vi "SP Format CH Traces.vi"(7 "Limit Traces":T5(array[cluster]), 8 "error in (no error)":errorcluster, 9 "CH2 Controls":T1={"Trace On"=TRUE, "Measure"=0, "Format"=0, "Autoscale"=TRUE, "Reference"=0.0, "\nRefUnit"="dB/Div", "Position"=5.0, "Scale"=10.0, "ScaleUnit"="dB/Div", "LimitOn"=TRUE, "LimitFill"=FALSE, "Display Data"=0, "Show Markers"=TRUE, "SXX"=""} {"Reference" format="%#.2g"; "Display Data" items=["Data", "Memory", "Data/Memory"]; "Format" items=["Log Mag", "Phase", "Expanded Phase", "Delay", "Smith", "Polar", "Lin Mag", "SWR", "Loss", "Real", "Imaginary"]; "Scale" min=0.001 step=1.0 format="%#.2g"; "Position" min=0.0 max=10.0}, 10 "CH1 Controls":T1={"Trace On"=TRUE, "Measure"=0, "Format"=0, "Autoscale"=TRUE, "Reference"=0.0, "\nRefUnit"="dB/Div", "Position"=5.0, "Scale"=10.0, "ScaleUnit"="dB/Div", "LimitOn"=TRUE, "LimitFill"=FALSE, "Display Data"=0, "Show Markers"=TRUE, "SXX"=""} {"Reference" format="%#.2g"; "Display Data" items=["Data", "Memory", "Data/Memory"]; "Format" items=["Log Mag", "Phase", "Expanded Phase", "Delay", "Smith", "Polar", "Lin Mag", "SWR", "Loss", "Real", "Imaginary"]; "Scale" min=0.001 step=1.0 format="%#.2g"; "Position" min=0.0 max=10.0}, 11 "Plot Reference":refnum<vi>) -> (0 "error out":errorcluster, 3 "Plot Reference":refnum<vi>)   [LabVIEW 2011]
uses:
  TypeDefs/SP Limit Type.ctl
  TypeDefs/SP Display Trace Controls.ctl
  TypeDefs/SP Display Format.ctl
  TypeDefs/SP Display Data.ctl
panel:
  # "Div"
  # "Div"
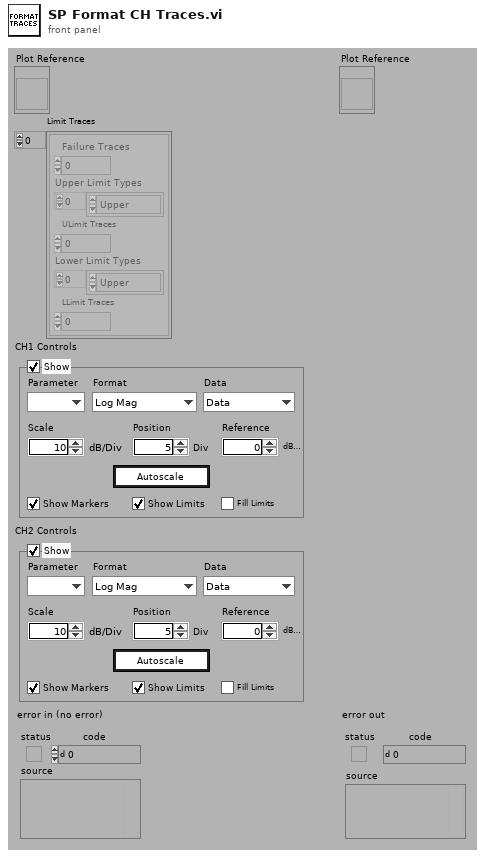
[diagram p1: front panel]
types:
  T1 = typedef "SP Display Trace Controls.ctl" = cluster{"Trace On":bool, "Measure":i32, "Format":T2, "Autoscale":bool, "Reference":dbl, "\nRefUnit":string, "Position":dbl, "Scale":dbl, "ScaleUnit":string, "LimitOn":bool, "LimitFill":bool, "Display Data":T3, "Show Markers":bool, "SXX":string}
  T2 = typedef "SP Display Format.ctl" = i32
  T3 = typedef "SP Display Data.ctl" = u16
  T4 = typedef "SP Limit Type.ctl" = enum16{"Upper", "Lower", "Delta", "Filter", "Referential"}
  T5 = cluster{"Failure Traces":i32, "Upper Limit Types":T4[], "ULimit Traces":i32, "Lower Limit Types":T4[], "LLimit Traces":i32}[]
  T6 = cluster{"Failure Traces":i32, "Upper Limit Types":T4[], "ULimit Traces":i32, "Lower Limit Types":T4[], "LLimit Traces":i32}
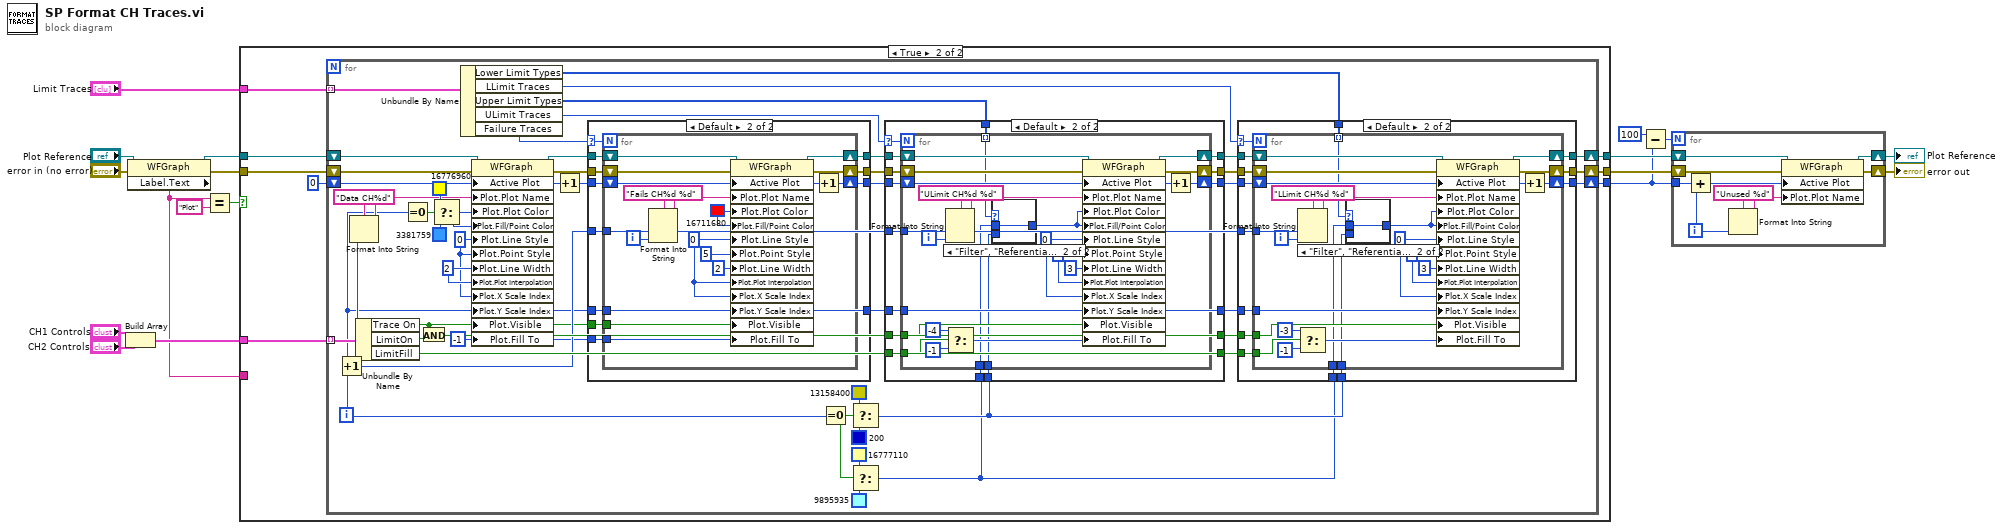
[diagram p0: block diagram]
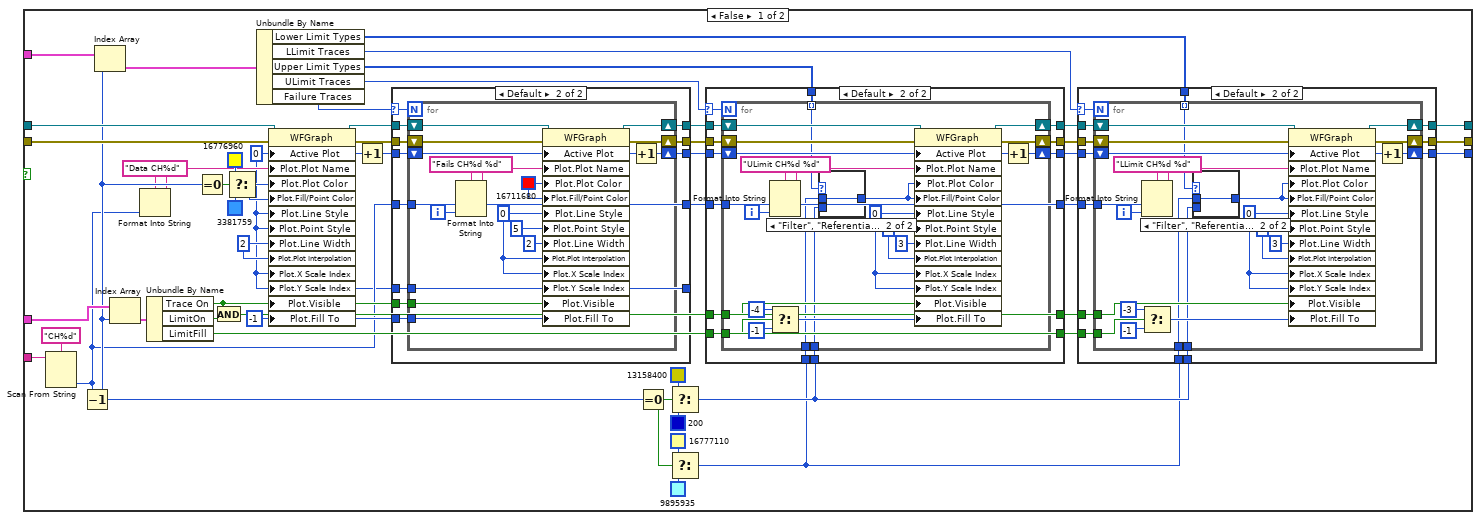
[diagram p2: hidden frame]
diagram:
  n1 = Build Array("CH1 Controls", "CH2 Controls") -> (w9:T1[])
  n2 = property on="Property Node" class="WFGraph"(reference="Plot Reference", error in="error in (no error)") -> (reference out=w14:refnum<vi>, error out=w16:errorcluster, "Label.Text"=w1:string)
  n3 = Equal?(x=w1, y="Plot") -> (x = y?=w12:bool)
  n4 = case shown="True" w12 {
    tunnel: [w50 w193] -> w7
    tunnel: [w51 w190] -> w8
    tunnel: "Limit Traces" -> [w67 w189]
    tunnel: w16 -> [w65 w192]
    tunnel: w14 -> [w64 w191]
    tunnel: w9 -> [w58 w187]
    tunnel: [w19 w186] -> w2
    tunnel: w1 -> [w41 _]
    frame False {
      w36 = i16 -1 ("Plot.Fill To")
      w59 = u8 2 ("Plot.Line Style")
      w21 = u32 0 ("Active Plot")
      n5 = Scan From String(format string="CH%d", input string=w41) -> (output 1=w33:i32)  [unwired: 2 in, 4 out]
      n6 = Decrement(x=w33) -> (x-1=w45:i32)
      n7 = Index Array(array=w67, index=w45) -> (element=w66:T6)
      n8 = Index Array(array=w58, index=w45) -> (element=w57:T1)
      n9 = Format Into String(format string="Data CH%d" ("Plot.Plot Name"), w33) -> (resulting string=w43:string)  [unwired: 2 in, 1 out]
      n10 = Unbundle By Name(w57) -> ("Trace On"=w37:bool, "LimitOn"=w56:bool, "LimitFill"=w48:bool)
      n11 = Equal To 0?(x=w45) -> (x = 0?=w61:bool)
      n12 = And(x=w37, y=w56) -> (x .and. y?=w47:bool)
      n13 = Select(t=u32 16776960, s=w61, f=u32 3381759) -> (s? t:f=w60:u32)
      n14 = Unbundle By Name(w66) -> ("Lower Limit Types"=w27:T4[], "LLimit Traces"=w52:i32, "Upper Limit Types"=w26:T4[], "ULimit Traces"=w55:i32, "Failure Traces"=w28:i32)
      n15 = property on="Property Node" class="WFGraph"(reference=w64, error in=w65, "Active Plot"=w21, "Plot.Plot Name"=w43, "Plot.Plot Color"=w60, "Plot.Fill/Point Color"=w60, "Plot.Line Style"=w21, "Plot.Point Style"=w21, "Plot.Line Width"=w59, "Plot.Plot Interpolation"=w59, "Plot.X Scale Index"=w21, "Plot.Y Scale Index"=w21, "Plot.Visible"=w37, "Plot.Fill To"=w36) -> (reference out=w30:refnum<vi>, error out=w29:errorcluster)
      n16 = Increment(x=w21) -> (x+1=w20:u32)
      n17 = case shown="Default" w28 {
        selector: w28 -> [_ w82]
        tunnel: [w74 w85] -> w38
        tunnel: [w73 w84] -> w39
        tunnel: [w72 w83] -> w40
        tunnel: w33 -> [w70 w76]
        tunnel: w20 -> [w74 w75]
        tunnel: w30 -> [w72 w81]
        tunnel: w29 -> [w73 w80]
        tunnel: w37 -> [_ w79]
        tunnel: w36 -> [_ w78]
        tunnel: w21 -> [w71 w77]
        tunnel: [w71 w77] -> _
        tunnel: [w70 w76] -> w32
        frame 0 {
        }
        frame Default {
          n18 = for {
            N: w82 -> [_]
            shift-right: [w100] -> w84
            shift-left: w80 -> [w101]
            shift-right: [w96] -> w83
            shift-left: w81 -> [w102]
            tunnel: w76 -> [w93]
            tunnel: w79 -> [w91]
            tunnel: w78 -> [w90]
            tunnel: w77 -> [w88]
            shift-right: [w86] -> w85
            shift-left: w75 -> [w87]
            i -> [w94]
            w92 = u32 16711680
            w89 = u8 0 ("Plot.Point Style")
            n19 = Format Into String(format string="Fails CH%d %d", w93, w94) -> (resulting string=w98:string)  [unwired: 2 in, 1 out]
            n20 = property on="Property Node" class="WFGraph"(reference=w102, error in=w101, "Active Plot"=w87, "Plot.Plot Name"=w98, "Plot.Plot Color"=w92, "Plot.Fill/Point Color"=w92, "Plot.Line Style"=w89, "Plot.Point Style"=u8 5 ("Plot.Line Style"), "Plot.Line Width"=u8 2, "Plot.Plot Interpolation"=w89, "Plot.X Scale Index"=w89, "Plot.Y Scale Index"=w88, "Plot.Visible"=w91, "Plot.Fill To"=w90) -> (reference out=w96:refnum<vi>, error out=w100:errorcluster)
            n21 = Increment(x=w87) -> (x+1=w86:u32)
          }
        }
      }
      n22 = Equal To 0?(x=w45) -> (x = 0?=w23:bool)
      n23 = Select(t=u32 13158400, s=w23, f=u32 200) -> (s? t:f=w49:u32)
      n24 = Select(t=u32 16777110, s=w23, f=u32 9895935) -> (s? t:f=w22:u32)
      n25 = case shown="Default" w55 {
        selector: w55 -> [_ w155]
        tunnel: [w147 w161] -> w46
        tunnel: [w148 w160] -> w54
        tunnel: [w146 w159] -> w53
        tunnel: w49 -> [_ w158]
        tunnel: w39 -> [w148 w157]
        tunnel: w40 -> [w146 w156]
        tunnel: w38 -> [w147 w149]
        tunnel: w47 -> [w145 w153]
        tunnel: w48 -> [w144 w154]
        tunnel: w32 -> [w143 w152]
        tunnel: [w144 w154] -> w35
        tunnel: [w145 w153] -> w34
        tunnel: [w143 w152] -> w31
        tunnel: w26 -> [_ w151]
        tunnel: w22 -> [_ w150]
        frame 0 {
        }
        frame Default {
          n26 = for {
            N: w155 -> [_]
            tunnel: w158 -> [w163]
            shift-right: [w181] -> w160
            shift-left: w157 -> [w182]
            shift-right: [w177] -> w159
            shift-left: w156 -> [w183]
            tunnel: w153 -> [w175]
            tunnel: w154 -> [w171]
            tunnel: w152 -> [w168]
            tunnel: w151 -> [w165] mode=indexing
            tunnel: w150 -> [w164]
            shift-right: [w166] -> w161
            shift-left: w149 -> [w167]
            i -> [w169]
            w178 = u8 2 ("Plot.Line Style")
            w170 = u8 0 ("Plot.Point Style")
            n27 = Format Into String(format string="ULimit CH%d %d", w168, w169) -> (resulting string=w179:string)  [unwired: 2 in, 1 out]
            n28 = Select(t=i16 -4, s=w171, f=i16 -1 ("Plot.Fill To")) -> (s? t:f=w173:i16)
            n29 = case shown="\"Filter\", \"Referential\"" w165 {
              tunnel: w164 -> [_ w185]
              tunnel: w163 -> [w184 _]
              tunnel: [w184 w185] -> w162
              frame "Upper".."Delta" {
              }
              frame "Filter", "Referential" {
              }
            }
            n30 = property on="Property Node" class="WFGraph"(reference=w183, error in=w182, "Active Plot"=w167, "Plot.Plot Name"=w179, "Plot.Plot Color"=w162, "Plot.Fill/Point Color"=w162, "Plot.Line Style"=w170, "Plot.Point Style"=w178, "Plot.Line Width"=u8 3, "Plot.Plot Interpolation"=w178, "Plot.X Scale Index"=w170, "Plot.Y Scale Index"=w170, "Plot.Visible"=w175, "Plot.Fill To"=w173) -> (reference out=w177:refnum<vi>, error out=w181:errorcluster)
            n31 = Increment(x=w167) -> (x+1=w166:u32)
          }
        }
      }
      n32 = case shown="Default" w52 {
        selector: w52 -> [_ w110]
        tunnel: [w104 w118] -> w19
        tunnel: [w105 w117] -> w50
        tunnel: [w103 w116] -> w51
        tunnel: w49 -> [_ w115]
        tunnel: w54 -> [w105 w114]
        tunnel: w53 -> [w103 w113]
        tunnel: w46 -> [w104 w106]
        tunnel: w34 -> [_ w112]
        tunnel: w35 -> [_ w111]
        tunnel: w31 -> [_ w109]
        tunnel: w27 -> [_ w108]
        tunnel: w22 -> [_ w107]
        frame 0 {
        }
        frame Default {
          n33 = for {
            N: w110 -> [_]
            tunnel: w115 -> [w121]
            shift-right: [w138] -> w117
            shift-left: w114 -> [w139]
            shift-right: [w134] -> w116
            shift-left: w113 -> [w140]
            tunnel: w112 -> [w132]
            tunnel: w111 -> [w128]
            tunnel: w109 -> [w125]
            tunnel: w108 -> [w120] mode=indexing
            tunnel: w107 -> [w122]
            shift-right: [w123] -> w118
            shift-left: w106 -> [w124]
            i -> [w126]
            w135 = u8 2 ("Plot.Line Style")
            w127 = u8 0 ("Plot.Point Style")
            n34 = Format Into String(format string="LLimit CH%d %d", w125, w126) -> (resulting string=w136:string)  [unwired: 2 in, 1 out]
            n35 = Select(t=i16 -3, s=w128, f=i16 -1 ("Plot.Fill To")) -> (s? t:f=w130:i16)
            n36 = case shown="\"Filter\", \"Referential\"" w120 {
              tunnel: w122 -> [_ w142]
              tunnel: w121 -> [w141 _]
              tunnel: [w141 w142] -> w119
              frame "Upper".."Delta" {
              }
              frame "Filter", "Referential" {
              }
            }
            n37 = property on="Property Node" class="WFGraph"(reference=w140, error in=w139, "Active Plot"=w124, "Plot.Plot Name"=w136, "Plot.Plot Color"=w119, "Plot.Fill/Point Color"=w119, "Plot.Line Style"=w127, "Plot.Point Style"=w135, "Plot.Line Width"=u8 3, "Plot.Plot Interpolation"=w135, "Plot.X Scale Index"=w127, "Plot.Y Scale Index"=w127, "Plot.Visible"=w132, "Plot.Fill To"=w130) -> (reference out=w134:refnum<vi>, error out=w138:errorcluster)
            n38 = Increment(x=w124) -> (x+1=w123:u32)
          }
        }
      }
    }
    frame True {
      n39 = for {
        shift-right: [w224] -> w193
        shift-left: w192 -> [w239]
        shift-right: [w223] -> w190
        shift-left: w191 -> [w238]
        tunnel: w189 -> [w233] mode=indexing
        shift-right: [w194] -> w186
        shift-left: u32 0 ("Active Plot") -> [w196]
        tunnel: w187 -> [w230] mode=indexing
        i -> [w207]
        w208 = i16 -1 ("Plot.Fill To")
        w231 = u32 0 ("Active Plot")
        w232 = u8 2 ("Plot.Line Style")
        n40 = Increment(x=w207) -> (x+1=w210:i32)
        n41 = Format Into String(format string="Data CH%d" ("Plot.Plot Name"), w210) -> (resulting string=w217:string)  [unwired: 2 in, 1 out]
        n42 = Unbundle By Name(w230) -> ("Trace On"=w209:bool, "LimitOn"=w229:bool, "LimitFill"=w219:bool)
        n43 = Equal To 0?(x=w207) -> (x = 0?=w235:bool)
        n44 = And(x=w209, y=w229) -> (x .and. y?=w220:bool)
        n45 = Select(t=u32 16776960, s=w235, f=u32 3381759) -> (s? t:f=w234:u32)
        n46 = Unbundle By Name(w233) -> ("Lower Limit Types"=w198:T4[], "LLimit Traces"=w222:i32, "Upper Limit Types"=w199:T4[], "ULimit Traces"=w228:i32, "Failure Traces"=w216:i32)
        n47 = property on="Property Node" class="WFGraph"(reference=w238, error in=w239, "Active Plot"=w196, "Plot.Plot Name"=w217, "Plot.Plot Color"=w234, "Plot.Fill/Point Color"=w234, "Plot.Line Style"=w231, "Plot.Point Style"=w231, "Plot.Line Width"=w232, "Plot.Plot Interpolation"=w232, "Plot.X Scale Index"=w231, "Plot.Y Scale Index"=w207, "Plot.Visible"=w209, "Plot.Fill To"=w208) -> (reference out=w212:refnum<vi>, error out=w211:errorcluster)
        n48 = Increment(x=w196) -> (x+1=w195:u32)
        n49 = case shown="Default" w216 {
          selector: w216 -> [_ w253]
          tunnel: [w245 w256] -> w215
          tunnel: [w244 w255] -> w213
          tunnel: [w243 w254] -> w214
          tunnel: w210 -> [_ w252]
          tunnel: w195 -> [w245 w246]
          tunnel: w212 -> [w243 w251]
          tunnel: w211 -> [w244 w250]
          tunnel: w209 -> [_ w249]
          tunnel: w208 -> [_ w248]
          tunnel: w207 -> [w242 w247]
          tunnel: [w242 w247] -> w206
          frame 0 {
          }
          frame Default {
            n50 = for {
              N: w253 -> [_]
              shift-right: [w271] -> w255
              shift-left: w250 -> [w272]
              shift-right: [w267] -> w254
              shift-left: w251 -> [w273]
              tunnel: w252 -> [w264]
              tunnel: w249 -> [w262]
              tunnel: w248 -> [w261]
              tunnel: w247 -> [w259]
              shift-right: [w257] -> w256
              shift-left: w246 -> [w258]
              i -> [w265]
              w263 = u32 16711680
              w260 = u8 0 ("Plot.Point Style")
              n51 = Format Into String(format string="Fails CH%d %d", w264, w265) -> (resulting string=w269:string)  [unwired: 2 in, 1 out]
              n52 = property on="Property Node" class="WFGraph"(reference=w273, error in=w272, "Active Plot"=w258, "Plot.Plot Name"=w269, "Plot.Plot Color"=w263, "Plot.Fill/Point Color"=w263, "Plot.Line Style"=w260, "Plot.Point Style"=u8 5 ("Plot.Line Style"), "Plot.Line Width"=u8 2, "Plot.Plot Interpolation"=w260, "Plot.X Scale Index"=w260, "Plot.Y Scale Index"=w259, "Plot.Visible"=w262, "Plot.Fill To"=w261) -> (reference out=w267:refnum<vi>, error out=w271:errorcluster)
              n53 = Increment(x=w258) -> (x+1=w257:u32)
            }
          }
        }
        n54 = Equal To 0?(x=w207) -> (x = 0?=w200:bool)
        n55 = Select(t=u32 13158400, s=w200, f=u32 200) -> (s? t:f=w221:u32)
        n56 = Select(t=u32 16777110, s=w200, f=u32 9895935) -> (s? t:f=w197:u32)
        n57 = case shown="Default" w228 {
          selector: w228 -> [_ w331]
          tunnel: [w321 w335] -> w225
          tunnel: [w320 w334] -> w227
          tunnel: [w319 w333] -> w226
          tunnel: w221 -> [_ w332]
          tunnel: w206 -> [w318 w328]
          tunnel: w220 -> [w317 w327]
          tunnel: w219 -> [w316 w326]
          tunnel: w210 -> [_ w330]
          tunnel: w215 -> [w321 w322]
          tunnel: w214 -> [w319 w329]
          tunnel: w213 -> [w320 w323]
          tunnel: [w318 w328] -> w205
          tunnel: [w317 w327] -> w203
          tunnel: [w316 w326] -> w204
          tunnel: w197 -> [_ w325]
          tunnel: w199 -> [_ w324]
          frame 0 {
          }
          frame Default {
            n58 = for {
              N: w331 -> [_]
              tunnel: w332 -> [w337]
              shift-right: [w356] -> w334
              shift-left: w323 -> [w357]
              shift-right: [w352] -> w333
              shift-left: w329 -> [w358]
              tunnel: w328 -> [w349]
              tunnel: w327 -> [w348]
              tunnel: w326 -> [w344]
              tunnel: w330 -> [w342]
              tunnel: w325 -> [w338]
              tunnel: w324 -> [w339] mode=indexing
              shift-right: [w340] -> w335
              shift-left: w322 -> [w341]
              i -> [w343]
              w353 = u8 2 ("Plot.Line Style")
              w350 = u8 0 ("Plot.Point Style")
              n59 = Format Into String(format string="ULimit CH%d %d", w342, w343) -> (resulting string=w354:string)  [unwired: 2 in, 1 out]
              n60 = Select(t=i16 -4, s=w344, f=i16 -1 ("Plot.Fill To")) -> (s? t:f=w346:i16)
              n61 = case shown="\"Filter\", \"Referential\"" w339 {
                tunnel: w338 -> [_ w360]
                tunnel: w337 -> [w359 _]
                tunnel: [w359 w360] -> w336
                frame "Upper".."Delta" {
                }
                frame "Filter", "Referential" {
                }
              }
              n62 = property on="Property Node" class="WFGraph"(reference=w358, error in=w357, "Active Plot"=w341, "Plot.Plot Name"=w354, "Plot.Plot Color"=w336, "Plot.Fill/Point Color"=w336, "Plot.Line Style"=w350, "Plot.Point Style"=w353, "Plot.Line Width"=u8 3, "Plot.Plot Interpolation"=w353, "Plot.X Scale Index"=w350, "Plot.Y Scale Index"=w349, "Plot.Visible"=w348, "Plot.Fill To"=w346) -> (reference out=w352:refnum<vi>, error out=w356:errorcluster)
              n63 = Increment(x=w341) -> (x+1=w340:u32)
            }
          }
        }
        n64 = case shown="Default" w222 {
          selector: w222 -> [_ w281]
          tunnel: [w275 w290] -> w194
          tunnel: [w276 w289] -> w224
          tunnel: [w274 w288] -> w223
          tunnel: w221 -> [_ w287]
          tunnel: w227 -> [w276 w286]
          tunnel: w226 -> [w274 w285]
          tunnel: w225 -> [w275 w277]
          tunnel: w205 -> [_ w284]
          tunnel: w203 -> [_ w283]
          tunnel: w204 -> [_ w282]
          tunnel: w210 -> [_ w280]
          tunnel: w198 -> [_ w279]
          tunnel: w197 -> [_ w278]
          frame 0 {
          }
          frame Default {
            n65 = for {
              N: w281 -> [_]
              tunnel: w287 -> [w292]
              shift-right: [w311] -> w289
              shift-left: w286 -> [w312]
              shift-right: [w307] -> w288
              shift-left: w285 -> [w313]
              tunnel: w284 -> [w304]
              tunnel: w283 -> [w303]
              tunnel: w282 -> [w299]
              tunnel: w280 -> [w297]
              tunnel: w279 -> [w293] mode=indexing
              tunnel: w278 -> [w294]
              shift-right: [w295] -> w290
              shift-left: w277 -> [w296]
              i -> [w298]
              w308 = u8 2 ("Plot.Line Style")
              w305 = u8 0 ("Plot.Point Style")
              n66 = Format Into String(format string="LLimit CH%d %d", w297, w298) -> (resulting string=w309:string)  [unwired: 2 in, 1 out]
              n67 = Select(t=i16 -3, s=w299, f=i16 -1 ("Plot.Fill To")) -> (s? t:f=w301:i16)
              n68 = case shown="\"Filter\", \"Referential\"" w293 {
                tunnel: w294 -> [_ w315]
                tunnel: w292 -> [w314 _]
                tunnel: [w314 w315] -> w291
                frame "Upper".."Delta" {
                }
                frame "Filter", "Referential" {
                }
              }
              n69 = property on="Property Node" class="WFGraph"(reference=w313, error in=w312, "Active Plot"=w296, "Plot.Plot Name"=w309, "Plot.Plot Color"=w291, "Plot.Fill/Point Color"=w291, "Plot.Line Style"=w305, "Plot.Point Style"=w308, "Plot.Line Width"=u8 3, "Plot.Plot Interpolation"=w308, "Plot.X Scale Index"=w305, "Plot.Y Scale Index"=w304, "Plot.Visible"=w303, "Plot.Fill To"=w301) -> (reference out=w307:refnum<vi>, error out=w311:errorcluster)
              n70 = Increment(x=w296) -> (x+1=w295:u32)
            }
          }
        }
      }
    }
  }
  n71 = Subtract(x=100, y=w2) -> (x-y=w3:u32)
  n72 = for {
    N: w3 -> [_]
    shift-right: [w366] -> w6
    shift-left: w8 -> [w368]
    shift-right: [w367] -> w5
    shift-left: w7 -> [w369]
    tunnel: w2 -> [w365]
    i -> [w363]
    n73 = Add(x=w365, y=w363) -> (x+y=w364:u32)
    n74 = Format Into String(format string="Unused %d" ("Plot.Plot Name"), w363) -> (resulting string=w361:string)  [unwired: 2 in, 1 out]
    n75 = property on="Property Node" class="WFGraph"(reference=w368, error in=w369, "Active Plot"=w364, "Plot.Plot Name"=w361) -> (reference out=w366:refnum<vi>, error out=w367:errorcluster)
  }
  "error out" <- w5
  "Plot Reference" <- w6
